vi "Main.vi"(11 "Module Admin":refnum<class "Delacor_lib_QMH_Module Admin.lvclass">) -> ()   [LabVIEW 2020, in "CML UI.lvlib"]
doc: "This template is based off of the Queued Message Handler design pattern and the Queued Message Handler project template that ships with LabVIEW.\n\nThe main difference is that the queue is private to this module and communication between modules is performed via Broadcast and Request events.\n\nRequest events are wrapped in public API methods and are handled in the Event Handling Loop (EHL) of this VI. Any module can register for Broadcast events sent by this module. The EHL generates messages based on user interface actions.\n\nThe Message Handling Loop (MHL) processes messages generated by the EHL, or by other messages. The messages are string values, so new messages can be added easily to the Message Cases case structure in the MHL. Each message cluster can also provide an optional value for Message Data, which is a variant that can be converted to whatever message-specific data is required.\n_____\nBased on DQMH Project Template 4.0.0.47.\n_____\nBased on DQMH Project Template 7.0.1.1316."
uses:
  CML UI.lvlib
  <vilib>/Delacor/Delacor QMH/Libraries/Module Admin_class/Delacor_lib_QMH_Module Admin.lvclass
  Module Data--cluster.ctl
  Configuration/Configuration--cluster.ctl
  Stop Argument--cluster.ctl
  <vilib>/Delacor/Delacor QMH/Libraries/Message Queue_class/Delacor_lib_QMH_Message Queue.lvclass/Delacor_lib_QMH_Message Queue.ctl
  <vilib>/Delacor/Delacor QMH/Libraries/Module Admin_class/Delacor_lib_QMH_Module Admin.lvclass/Delacor_lib_QMH_Module Admin.ctl
  Configuration/Configuration.lvclass
  Configuration/Configuration.lvclass/Configuration.ctl
  <vilib>/Delacor/Delacor QMH/Libraries/Message Queue_class/Delacor_lib_QMH_Enqueue Message (Single).vi
  <vilib>/Delacor/Delacor QMH/Libraries/Module Admin_class/Delacor_lib_QMH_Get External Launch.vi
  Configuration/Get Configuration.vi
  <vilib>/Delacor/Delacor QMH/Libraries/Message Queue_class/Delacor_lib_QMH_Message Queue.lvclass
  Settings Editor/Settings Editor.lvlib
  Acquisition/Acquisition.lvlib
  Logger/Logger.lvlib
  <vilib>/Peloton/Peloton Config/DCFG Framework/Peloton_lib_DCFG Framework.lvlib
  CML Shared/CML Shared.lvlib
  <vilib>/Peloton/Peloton Config/DCFG Framework/Configuration_class/Configuration.lvclass
panel:
  in  "About DQMH":bool
  out "Logger Running?":bool
  out "Settings Editor Running?":bool
  out "Acquisition Running?":bool
  out "Data":waveform(dbl)[](graph)
  out "Calibrated?":bool
  in  "Calibrate":bool
  in  "Settings":bool
  in  "Start":bool
  in  "Stop":bool
  out "error out":errorcluster
  out "Status":string
  out "version":string
  # "Continuous Measurement Data Logger"
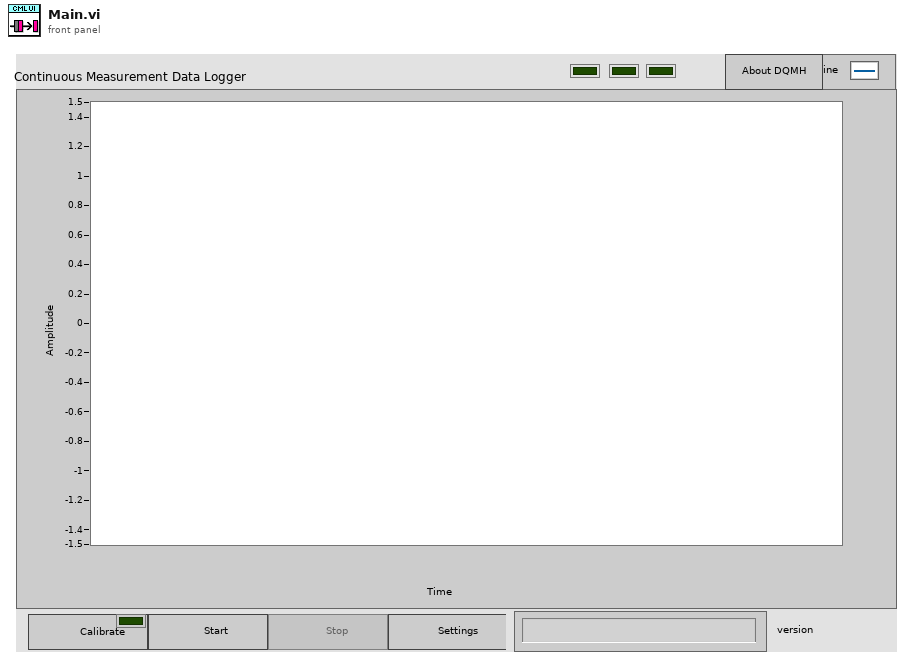
[diagram p1: front panel]
types:
  T1 = typedef "CML UI.lvlib/Request Events--cluster.ctl" = cluster{"Stop Module":refnum<user-event>, "Show Panel":refnum<user-event>, "Hide Panel":refnum<user-event>, "Get Module Execution Status":refnum<user-event>, "Show Diagram":refnum<user-event>}
  T2 = typedef "Settings Editor.lvlib/Broadcast Events--cluster.ctl" = cluster{"Module Did Init":refnum<user-event>, "Status Updated":refnum<user-event>, "Error Reported":refnum<user-event>, "Module Did Stop":refnum<user-event>, "Update Module Execution Status":refnum<user-event>, "Application Settings Updated":refnum<user-event>}
  T3 = typedef "Acquisition.lvlib/Broadcast Events--cluster.ctl" = cluster{"Module Did Init":refnum<user-event>, "Status Updated":refnum<user-event>, "Error Reported":refnum<user-event>, "Module Did Stop":refnum<user-event>, "Update Module Execution Status":refnum<user-event>, "Acquisition Started":refnum<user-event>, "Acquisition Stopped":refnum<user-event>, "Data Updated":refnum<user-event>, "Device Calibrated":refnum<user-event>}
  T4 = typedef "Logger.lvlib/Broadcast Events--cluster.ctl" = cluster{"Module Did Init":refnum<user-event>, "Status Updated":refnum<user-event>, "Error Reported":refnum<user-event>, "Module Did Stop":refnum<user-event>, "Update Module Execution Status":refnum<user-event>, "Logging Stopped":refnum<user-event>, "File Initialized":refnum<user-event>}
  T5 = typedef "Peloton_lib_DCFG Framework.lvlib/Broadcast Events--cluster.ctl" = cluster{"Module Did Init":refnum<user-event>, "Status Updated":refnum<user-event>, "Error Reported":refnum<user-event>, "Module Did Stop":refnum<user-event>, "Update Module Execution Status":refnum<user-event>, "View Changed":refnum<user-event>, "Main Window Closed":refnum<user-event>, "Configuration Committed":refnum<user-event>, "Configuration Canceled":refnum<user-event>, "Views List Updated":refnum<user-event>, "Config Folder Path Updated":refnum<user-event>}
  T6 = typedef "CML UI.lvlib/Module Data--cluster.ctl" = cluster{"Status":string, "Start Ref":refnum<vi>, "Settings Ref":refnum<vi>, "Stop Ref":refnum<vi>, "Status Ref":refnum<vi>, "Data Ref":refnum<vi>, "Configuration":T7}
  T7 = typedef "CML UI.lvlib/Configuration.lvclass/Configuration--cluster.ctl" = cluster{"test1":dbl, "test2":dbl}
  T8 = enum32{"invalid lock state", "Not Locked", "Locked (No Password)", "Password-protected"}
  T9 = typedef "CML UI.lvlib/Stop Argument--cluster.ctl" = cluster{"Origin":string, "Exit via Stop Module Req?":bool, "Wait for Module to stop?":bool}
  T10 = enum32{"Invalid", "Standard", "Closed", "Hidden", "Minimized", "Maximized"}
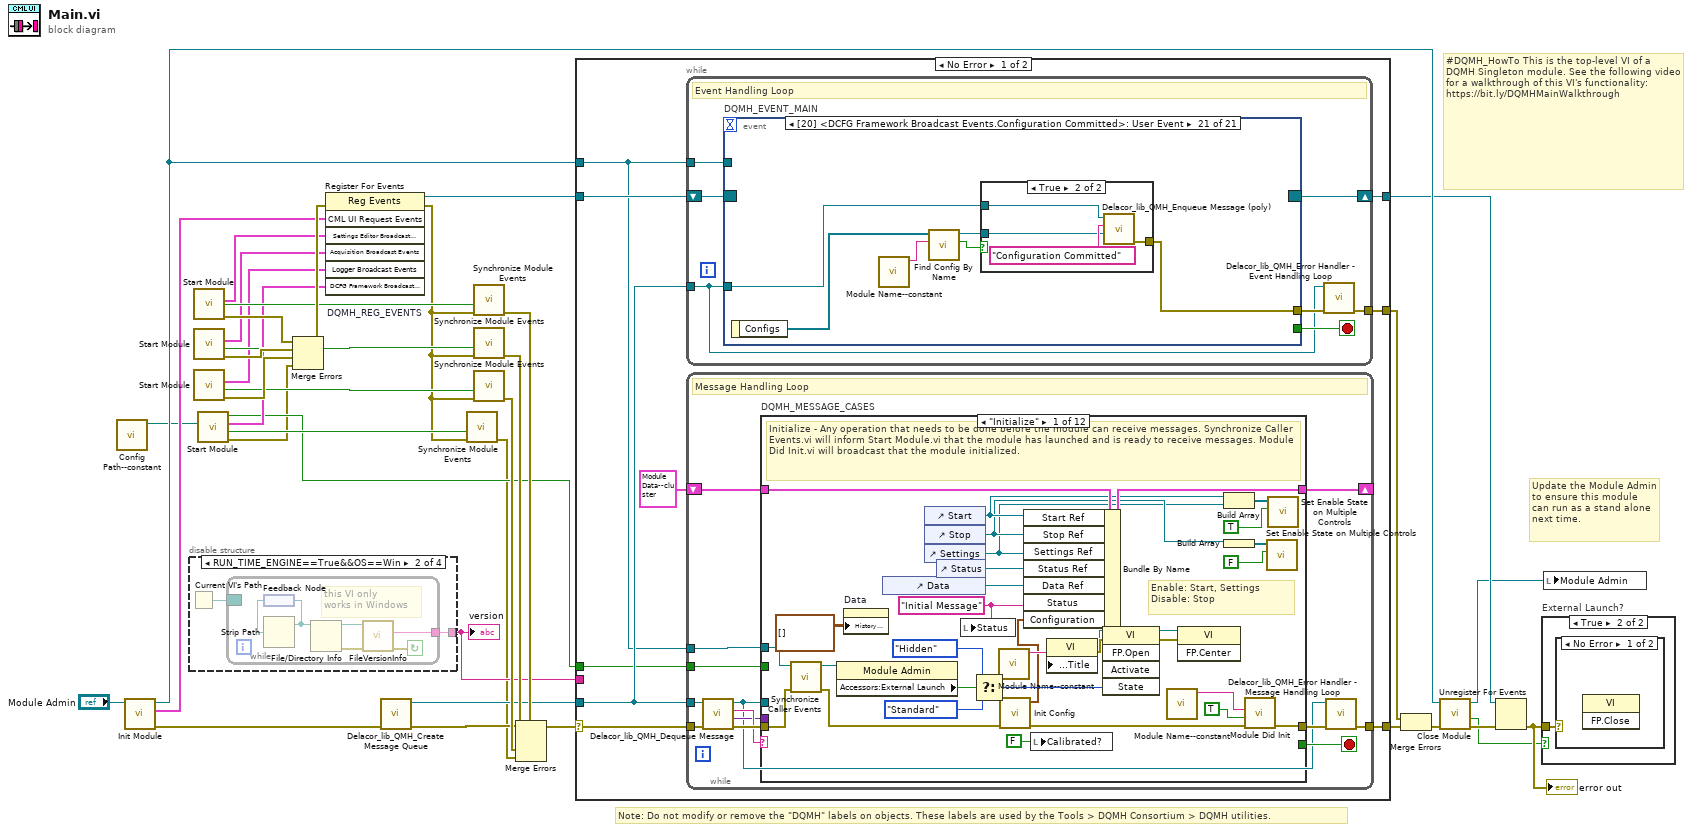
[diagram p0: block diagram]
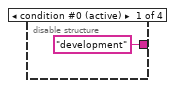
[diagram p2: hidden frame]
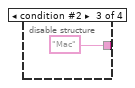
[diagram p3: hidden frame]
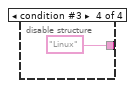
[diagram p4: hidden frame]
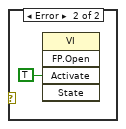
[diagram p6: hidden frame]
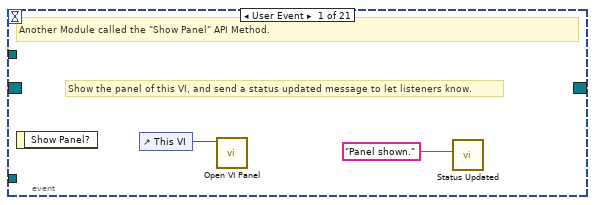
[diagram p7: hidden frame]
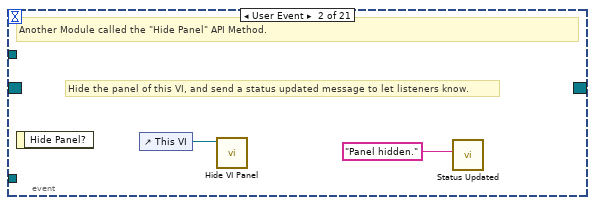
[diagram p8: hidden frame]
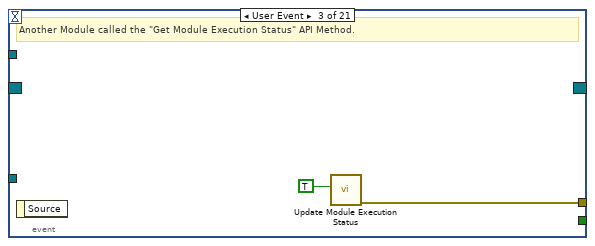
[diagram p9: hidden frame]
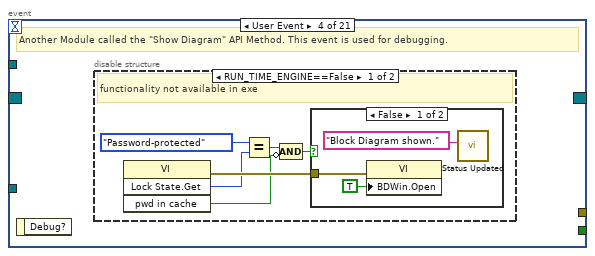
[diagram p10: hidden frame]
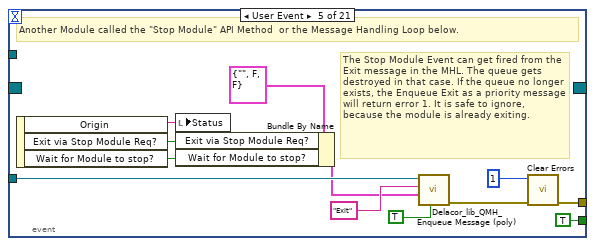
[diagram p13: hidden frame]
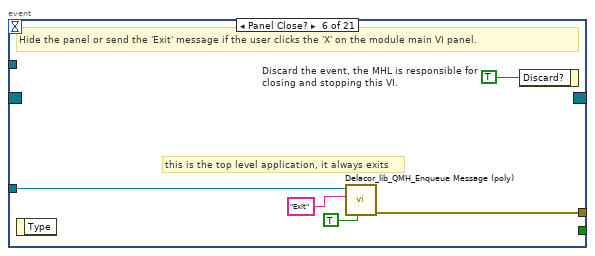
[diagram p14: hidden frame]
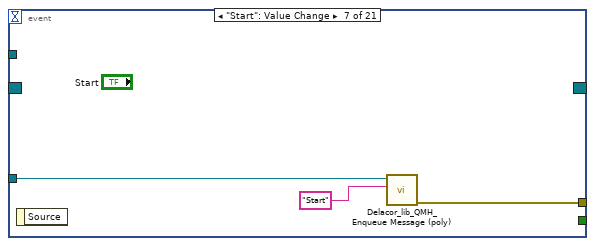
[diagram p15: hidden frame]
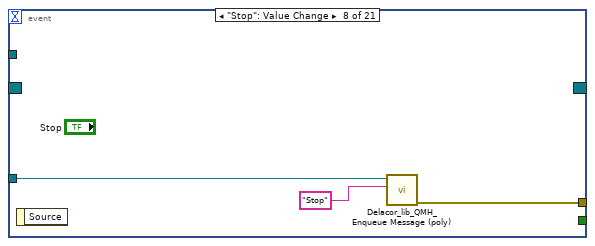
[diagram p16: hidden frame]
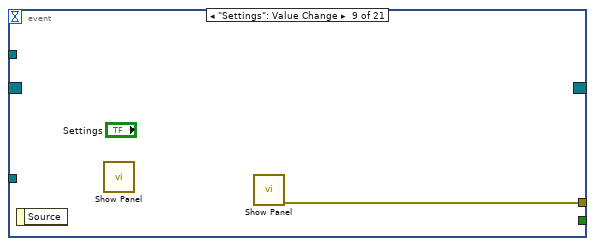
[diagram p17: hidden frame]
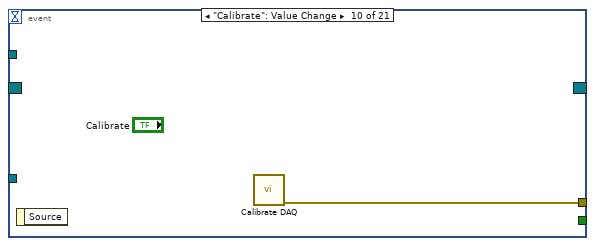
[diagram p18: hidden frame]
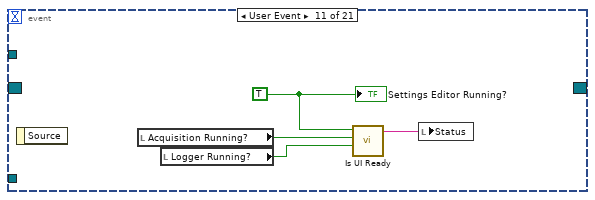
[diagram p19: hidden frame]
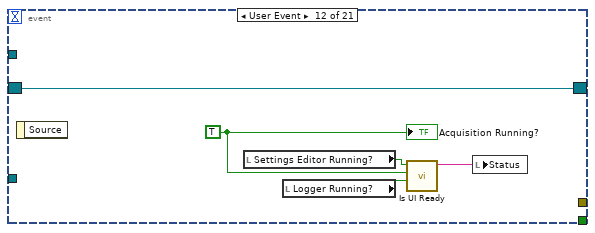
[diagram p20: hidden frame]
diagram:
  # "#DQMH_HowTo This is the top-level VI of a DQMH Singleton module. See the following video for a walkthrough of this VI's functionality: https://bit.ly/DQMHMainWalkthrough"
  # "Note: Do not modify or remove the \"DQMH\" labels on objects. These labels are used by the Tools > DQMH Consortium > DQMH utilities."
  # "Update the Module Admin to ensure this module can run as a stand alone next time."
  n1 = call "Config Path--constant.vi"() -> ("File Path"=w1:path)  [unwired: 11 in]
  n2 = call "Init Module.vi"("Singleton Module Admin in"="Module Admin") -> ("error out"=w35:errorcluster, "CML UI Request Events"=w19:T1, "Singleton Module Admin out"=w22:refnum<class "Delacor_lib_QMH_Module Admin.lvclass">)  [unwired: 8 in]
  n3 = disable-structure "Conditional Disable Structure" shown="RUN_TIME_ENGINE==True&&OS==Win" {
    disable-tunnel: ["development" w39 "Mac" "Linux"] -> w8
    frame condition #0 (active) {
    }
    frame condition #1 {
      n4 = Current VI's Path() -> (path=w40:path)
      n5 = while {
        border: w40 -> [_]
        tunnel: [w41] -> w39
        stop <- w45 continue-if-true
        # "this VI only \nworks in Windows"
        n6 = feedback #1() -> (w44:path)
        n7 = Strip Path(path=w44) -> (stripped path=w43:path)  [unwired: 1 out]
        n8 = feedback-in #1(w43) -> ()
        n9 = File/Directory Info(path=w43) -> (path out=w42:path, error out=w46:errorcluster)  [unwired: 1 in, 5 out]
        n10 = call <vilib>:"FileVersionInfo.vi"("error in (no error)"=w46, "Application Path in"=w42) -> ("error out"=w45:errorcluster, "File Version Info"=w41:string)  [unwired: 6 in, 2 out]
      }
    }
    frame condition #2 {
    }
    frame condition #3 {
    }
  }
  "version" <- w8
  n11 = call <vilib>:"Start Module.vi"() -> ("error out"=w26:errorcluster, "Wait for Event Sync?"=w14:bool, "Settings Editor Broadcast Events"=w13:T2)  [unwired: 8 in, 1 out]
  n12 = call <vilib>:"Start Module.vi"() -> ("error out"=w25:errorcluster, "Wait for Event Sync?"=w11:bool, "Acquisition Broadcast Events"=w12:T3)  [unwired: 8 in, 1 out]
  n13 = call <vilib>:"Start Module.vi"() -> ("error out"=w24:errorcluster, "Wait for Event Sync?"=w9:bool, "Logger Broadcast Events"=w10:T4)  [unwired: 8 in, 1 out]
  n14 = call <vilib>:"Start Module.vi"("Config Folder"=w1) -> ("error out"=w4:errorcluster, "Wait for Event Sync?"=w6:bool, "DCFG Framework Broadcast Events"=w7:T5, "Module Was Already Running?"=w5:bool)  [unwired: 7 in]
  n15 = Merge Errors(w26, w25, w24, w4) -> (w23:errorcluster)
  n16 = register-events "DQMH_REG_EVENTS"(error in=w23, w19, w13, w12, w10, w7) -> (reference out=w20:refnum<event-registration>, error out=w3:errorcluster)  [unwired: 1 in]
  n17 = call <vilib>:"Delacor_lib_QMH_Create Message Queue.vi"("error in"=w35) -> ("error out"=w30:errorcluster, "Message Queue"=w18:refnum<class "Delacor_lib_QMH_Message Queue.lvclass">)  [unwired: 9 in]
  n18 = call <vilib>:"Synchronize Module Events.vi"("error in (no error)"=w3, "Wait for Event Sync?"=w6) -> ("error out"=w2:errorcluster)  [unwired: 9 in]
  n19 = call <vilib>:"Synchronize Module Events.vi"("error in"=w3, "Wait for Event Sync?"=w14) -> ("error out"=w28:errorcluster)  [unwired: 9 in]
  n20 = call <vilib>:"Synchronize Module Events.vi"("error in"=w3, "Wait for Event Sync?"=w11) -> ("error out"=w27:errorcluster)  [unwired: 9 in]
  n21 = call <vilib>:"Synchronize Module Events.vi"("error in"=w3, "Wait for Event Sync?"=w9) -> ("error out"=w37:errorcluster)  [unwired: 9 in]
  n22 = Merge Errors(w30, w28, w27, w37, w2) -> (w29:errorcluster)
  n23 = case shown="No Error" w29 {
    selector: w29 -> [w55 w292]
    tunnel: [w57 w291] -> w36
    tunnel: [w54 w290] -> w21
    tunnel: w20 -> [w52 w290]
    tunnel: w18 -> [w51 w283]
    tunnel: [w56 _] -> w33
    tunnel: w22 -> [w50 w286]
    tunnel: w8 -> [_ _]
    tunnel: w5 -> [w49 w282]
    frame No Error {
      n24 = while {
        tunnel: w51 -> [w58]
        shift-right: [w61] -> w54
        shift-left: w52 -> [w62]
        tunnel: [w63] -> w56
        tunnel: w50 -> [w59]
        stop <- w60 stop-if-true
        # "Event Handling Loop"
        n25 = event "DQMH_EVENT_MAIN" shown="[20] <DCFG Framework Broadcast Events.Configuration Committed>: User Event" {
          selector: w62 -> [_ _ _ _ _ _ _ _ _ _ _ w113 _ _ _ _ _ _ _ _ _]
          dyn-events: [_ _ _ _ _ _ _ _ _ _ _ w113 _ _ _ _ _ _ _ _ _] -> w61
          timeout: _ -> [_ _ _ _ _ _ _ _ _ _ _ _ _ _ _ _ _ _ _ _ _]
          tunnel: [_ _ _ _ TRUE ("Discard?") _ _ _ _ _ _ _ _ _ _ _ _ _ _ _ _] -> w60
          tunnel: w58 -> [_ _ _ _ w87 w94 w97 w100 _ _ _ _ _ _ _ w125 w127 _ _ _ w134]
          tunnel: [_ _ w70 _ w90 w96 w99 w102 w103 w104 _ _ _ _ w123 _ _ _ _ w130 w136] -> w64
          tunnel: w59 -> [_ _ _ _ _ _ _ _ _ _ _ _ _ _ _ _ _ _ _ _ _]
          event User Event {
            # "Show the panel of this VI, and send a status updated message to let listeners know."
            # "Another Module called the \"Show Panel\" API Method."
            n26 = event-data() -> ()  [unwired: 1 in, 1 out]
            n27 = control-ref of="This VI"() -> (w66:refnum<vi>)
            n28 = call "Open VI Panel.vi"("VI"=w66) -> ()  [unwired: 10 in, 1 out]
            n29 = call "Status Updated.vi"("Status"="Panel shown." ("format string")) -> ()  [unwired: 10 in, 1 out]
          }
          event User Event {
            # "Hide the panel of this VI, and send a status updated message to let listeners know."
            # "Another Module called the \"Hide Panel\" API Method."
            n30 = event-data() -> ()  [unwired: 1 in, 1 out]
            n31 = control-ref of="This VI"() -> (w68:refnum<vi>)
            n32 = call "Hide VI Panel.vi"("VI"=w68) -> ()  [unwired: 10 in, 1 out]
            n33 = call "Status Updated.vi"("Status"="Panel hidden." ("format string")) -> ()  [unwired: 10 in, 1 out]
          }
          event User Event {
            # "Another Module called the \"Get Module Execution Status\" API Method."
            n34 = event-data() -> ()  [unwired: 1 in, 1 out]
            n35 = call "Update Module Execution Status.vi"("Running?"=TRUE) -> ("error out"=w70:errorcluster)  [unwired: 10 in]
          }
          event User Event {
            # "Another Module called the \"Show Diagram\" API Method. This event is used for debugging."
            n36 = event-data() -> ()  [unwired: 1 in, 1 out]
            n37 = disable-structure shown="RUN_TIME_ENGINE==False" {
              frame condition #0 (active) {
                # "functionality not available in exe"
                n38 = invoke on="Invoke Node" class="VI" method="Lock State.Get"() -> (error out=w76:errorcluster, "Get Lock State"=w75:T8, "pwd in cache"=w72:bool)  [unwired: 4 in, 1 out]
                n39 = Equal?(x=T8."Password-protected", y=w75) -> (x = y?=w73:bool)
                n40 = Compound Arithmetic op=AND(w73, invert w72) -> (w71:bool)
                n41 = case shown="False" w71 {
                  tunnel: w76 -> [w79 _]
                  frame False {
                    n42 = property on="Property Node" class="VI"(error in=w79, "BDWin.Open"=TRUE ("Block Diagram Window:Open")) -> ()  [unwired: 1 in, 2 out]
                    n43 = call "Status Updated.vi"("Status"="Block Diagram shown." ("format string")) -> ()  [unwired: 10 in, 1 out]
                  }
                  frame True {
                    # "Password-protected VI, and the password is not in the cache. Do not show the diagram."
                  }
                }
              }
              frame condition #1 {
              }
            }
          }
          event User Event {
            # "The Stop Module Event can get fired from the Exit message in the MHL. The queue gets destroyed in that case. If the queue no longer exists, the Enqueue Exit as a priority message will return error 1. It is safe to ignore, because the module is already exiting."
            # "Another Module called the \"Stop Module\" API Method  or the Message Handling Loop below."
            n44 = event-data() -> ("Origin"=w86:string, "Exit via Stop Module Req?"=w82:bool, "Wait for Module to stop?"=w81:bool)  [unwired: 1 in]
            n45 = local write "Status"(w86) -> ()
            n46 = Bundle By Name(cluster=T9 {"Origin"="", "Exit via Stop Module Req?"=FALSE, "Wait for Module to stop?"=FALSE} ("Stop Argument"), "Exit via Stop Module Req?"=w82, "Wait for Module to stop?"=w81) -> (w80:T9)
            n47 = call-poly <vilib>:"Delacor_lib_QMH_Enqueue Message (poly).vi"("Priority Message? (F)"=TRUE, "Message Data"=w80, "Message"="Exit", "Message Queue in"=w87) -> ("error out"=w91:errorcluster)  [unwired: 6 in, 1 out]
            n48 = call <vilib>:"Clear Errors.vi"("error in (no error)"=w91, "specific error code to clear (0: all)"=1) -> ("error out"=w90:errorcluster)  [unwired: 4 in, 1 out]
          }
          event Panel Close? {
            w95 = TRUE  # Discard the event, the MHL is responsible for closing and stopping this VI.
            # "this is the top level application, it always exits"
            # "Hide the panel or send the 'Exit' message if the user clicks the 'X' on the module main VI panel."
            n49 = event-data() -> ()  [unwired: 1 in, 1 out]
            n50 = call-poly <vilib>:"Delacor_lib_QMH_Enqueue Message (poly).vi"("Priority Message? (F)"=TRUE, "Message"="Exit", "Message Queue in"=w94) -> ("error out"=w96:errorcluster)  [unwired: 7 in, 1 out]
            n51 = event-data ("Event Filter Node")("Discard?"=w95) -> ()  [unwired: 1 in, 1 out]
          }
          event "Start": Value Change {
            n52 = event-data() -> ()  [unwired: 1 in, 1 out]
            n53 = call-poly <vilib>:"Delacor_lib_QMH_Enqueue Message (poly).vi"("Message"="Start", "Message Queue in"=w97) -> ("error out"=w99:errorcluster)  [unwired: 8 in, 1 out]
          }
          event "Stop": Value Change {
            n54 = event-data() -> ()  [unwired: 1 in, 1 out]
            n55 = call-poly <vilib>:"Delacor_lib_QMH_Enqueue Message (poly).vi"("Message"="Stop", "Message Queue in"=w100) -> ("error out"=w102:errorcluster)  [unwired: 8 in, 1 out]
          }
          event "Settings": Value Change {
            n56 = event-data() -> ()  [unwired: 1 in, 1 out]
            n57 = call <vilib>:"Show Panel.vi"() -> ()  [unwired: 11 in, 1 out]
            n58 = call <vilib>:"Show Panel.vi"() -> ("error out"=w103:errorcluster)  [unwired: 11 in]
          }
          event "Calibrate": Value Change {
            n59 = event-data() -> ()  [unwired: 1 in, 1 out]
            n60 = call "Calibrate DAQ.vi"() -> ("error out"=w104:errorcluster)  [unwired: 11 in]
          }
          event User Event {
            w106 = TRUE ("Settings Editor Running?")
            n61 = event-data() -> ()  [unwired: 1 in, 1 out]
            n62 = local read "Acquisition Running?"() -> (w108:bool)
            n63 = local read "Logger Running?"() -> (w107:bool)
            n64 = call "Is UI Ready.vi"("Logger Running?"=w107, "Acquisition Running?"=w108, "Settings Editor Running?"=w106) -> ("Status"=w105:string)  [unwired: 8 in]
            n65 = local write "Status"(w105) -> ()
            "Settings Editor Running?" <- w106
          }
          event User Event {
            w111 = TRUE ("Acquisition Running?")
            n66 = event-data() -> ()  [unwired: 1 in, 1 out]
            n67 = local read "Settings Editor Running?"() -> (w110:bool)
            n68 = local read "Logger Running?"() -> (w109:bool)
            n69 = call "Is UI Ready.vi"("Logger Running?"=w109, "Acquisition Running?"=w111, "Settings Editor Running?"=w110) -> ("Status"=w112:string)  [unwired: 8 in]
            n70 = local write "Status"(w112) -> ()
            "Acquisition Running?" <- w111
          }
          event User Event {
            w116 = TRUE ("Logger Running?")
            n71 = event-data() -> ()  [unwired: 1 in, 1 out]
            n72 = local read "Settings Editor Running?"() -> (w115:bool)
            n73 = local read "Acquisition Running?"() -> (w114:bool)
            n74 = call "Is UI Ready.vi"("Logger Running?"=w116, "Acquisition Running?"=w114, "Settings Editor Running?"=w115) -> ("Status"=w117:string)  [unwired: 8 in]
            n75 = local write "Status"(w117) -> ()
            "Logger Running?" <- w116
          }
          event User Event {
            n76 = event-data() -> ("Status"=w118:string)  [unwired: 1 in]
            "Status" <- w118
            n77 = call "Status Updated.vi"("Status"=w118) -> ()  [unwired: 10 in, 1 out]
          }
          event User Event {
            n78 = event-data() -> ("Error"=w123:errorcluster, "Module Name"=w121:string)  [unwired: 1 in]
            n79 = Unbundle By Name(w123) -> ("code"=w122:i32)
            n80 = Format Into String(format string="Error %d at %s", w122, w121) -> (resulting string=w120:string)  [unwired: 2 in, 1 out]
            n81 = local write "Status"(w120) -> ()
          }
          event User Event {
            n82 = event-data() -> ()  [unwired: 1 in, 1 out]
            n83 = call-poly <vilib>:"Delacor_lib_QMH_Enqueue Message (poly).vi"("Message"="Acquisition Started Interlocks", "Message Queue in"=w125) -> ()  [unwired: 8 in, 2 out]
          }
          event User Event {
            n84 = event-data() -> ()  [unwired: 1 in, 1 out]
            n85 = call-poly <vilib>:"Delacor_lib_QMH_Enqueue Message (poly).vi"("Message"="Acquisition Stopped Interlocks", "Message Queue in"=w127) -> ()  [unwired: 8 in, 2 out]
          }
          event User Event {
            n86 = event-data() -> ("Graph Data"=→"Data":waveform(dbl)[])  [unwired: 1 in]
          }
          event User Event {
            n87 = event-data() -> ()  [unwired: 1 in, 1 out]
            "Calibrated?" <- TRUE ("Calibrated?")
          }
          event "About DQMH": Value Change {
            # "Display the About DQMH box"
            n88 = event-data() -> ()  [unwired: 1 in, 1 out]
            n89 = call <vilib>:"DQMH_About Box.vi"() -> ("error out"=w130:errorcluster)  [unwired: 11 in]
          }
          event User Event {
            n90 = event-data() -> ("Configs"=w135:refnum<class "Configuration.lvclass">[])  [unwired: 1 in]
            n91 = call "Module Name--constant.vi"() -> ("Module Name"=w133:string)  [unwired: 11 in]
            n92 = call <vilib>:"Find Config By Name.vi"("Config Name"=w133, "All Config Classes"=w135) -> ("Found"=w132:bool, "Configuration"=w131:refnum<class "Configuration.lvclass">)  [unwired: 6 in, 2 out]
            n93 = case shown="True" w132 {
              tunnel: w134 -> [_ w139]
              tunnel: [_ w140] -> w136
              tunnel: w131 -> [_ w137]
              frame False {
              }
              frame True {
                n94 = call-poly <vilib>:"Delacor_lib_QMH_Enqueue Message (poly).vi"("Message Data"=w137, "Message"="Configuration Committed", "Message Queue in"=w139) -> ("error out"=w140:errorcluster)  [unwired: 7 in, 1 out]
              }
            }
          }
        }
        n95 = call-dynamic "Delacor_lib_QMH_Error Handler - Event Handling Loop.vi"("error in"=w64, "Message Queue in"=w58) -> ("dup error in"=w63:errorcluster)  [unwired: 8 in, 1 out]
      }
      n96 = while {
        tunnel: w51 -> [w144]
        shift-right: [w148] -> _
        shift-left: T6 {"Status"="", "Start Ref"=refnum, "Settings Ref"=refnum, "Stop Ref"=refnum, "Status Ref"=refnum, "Data Ref"=refnum, "Configuration"={"test1"=0.0, "test2"=0.0}} ("Data Cluster") -> [w149]
        tunnel: w55 -> [w152]
        tunnel: [w150] -> w57
        tunnel: w50 -> [w142]
        tunnel: w49 -> [w141]
        stop <- w147 stop-if-true
        # "Message Handling Loop"
        n97 = call-dynamic "Delacor_lib_QMH_Dequeue Message.vi"("error in"=w152, "Message Queue in"=w144) -> ("error out"=w151:errorcluster, "Message Data"=w145:variant, "Message"=w146:string, "Message Queue out"=w143:refnum<class "Delacor_lib_QMH_Message Queue.lvclass">)  [unwired: 6 in]
        n98 = case "DQMH_MESSAGE_CASES" shown="\"Initialize\"" w146 {
          selector: w146 -> [_ _ _ _ _ _ _ _ _ _ w268 _]
          tunnel: w143 -> [_ _ _ _ _ _ _ _ w221 w249 _ _]
          tunnel: w151 -> [w183 w187 w190 w200 w203 w213 w216 w218 w229 w257 w271 w280]
          tunnel: [w182 w187 w189 w200 w202 w213 w215 w218 w225 w250 w272 w277] -> w153
          tunnel: w149 -> [w173 w186 w188 w192 w201 w205 w214 w217 w223 w248 w269 w279]
          tunnel: [w165 w186 w188 w192 w201 w205 w214 w217 w223 w248 w269 w278] -> w148
          tunnel: [_ _ _ _ _ _ _ _ _ w247 _ _] -> w147
          tunnel: w145 -> [_ _ _ _ _ _ _ _ w222 w246 _ w276]
          tunnel: w142 -> [w174 _ _ _ _ _ _ _ w220 w241 _ _]
          tunnel: w141 -> [_ _ _ _ _ _ _ _ _ w237 _ _]
          frame "Initialize" {
            w168 = "Initial Message" ("Initial Message")
            # "Enable: Start, Settings\nDisable: Stop"
            # "Initialize - Any operation that needs to be done before the module can receive messages. Synchronize Caller Events.vi will inform Start Module.vi that the module has launched and is ready to receive messages. Module Did Init.vi will broadcast that the module initialized."
            n99 = call "Synchronize Caller Events.vi"("error in"=w183, "Singleton Module Admin in"=w174) -> ("error out"=w156:errorcluster, "Singleton Module Admin out"=w170:refnum<class "Delacor_lib_QMH_Module Admin.lvclass">)  [unwired: 8 in]
            n100 = property on="Property Node" class="Module Admin"(reference=w170) -> ("Accessors:External Launch"=w178:bool)  [unwired: 1 in, 2 out]
            n101 = property on="Data" class="WFChart (strict)"("History Data"=waveform(dbl)[][] []) -> ()  [unwired: 2 in, 2 out]
            n102 = control-ref of="Data"() -> (w166:refnum<vi>)
            n103 = control-ref of="Start"() -> (w159:refnum<vi>)
            n104 = control-ref of="Stop"() -> (w158:refnum<vi>)
            n105 = control-ref of="Settings"() -> (w157:refnum<vi>)
            n106 = control-ref of="Status"() -> (w167:refnum<vi>)
            n107 = local write "Status"(w168) -> ()
            n108 = Select(t=T10."Hidden" ("State"), s=w178, f=T10."Standard" ("State")) -> (s? t:f=w175:T10)
            n109 = call "Module Name--constant.vi"() -> ("Module Name"=w181:string)  [unwired: 11 in]
            n110 = call "Init Config.vi"("error in"=w156) -> ("error out"=w155:errorcluster, "Configuration"=w154:T7)  [unwired: 9 in]
            n111 = Bundle By Name(cluster=w173, "Start Ref"=w159, "Stop Ref"=w158, "Settings Ref"=w157, "Status Ref"=w167, "Data Ref"=w166, "Status"=w168, "Configuration"=w154) -> (w165:T6)
            n112 = local write "Calibrated?"(FALSE ("Calibrated?")) -> ()
            n113 = property on="Property Node" class="VI"("Front Panel.Title"=w181) -> (reference out=w180:refnum<vi>, error out=w185:errorcluster)  [unwired: 2 in]
            n114 = invoke on="Invoke Node" class="VI" method="FP.Open"(reference=w180, error in=w185, "State"=w175) -> (reference out=w179:refnum<vi>, error out=w184:errorcluster)  [unwired: 2 in, 3 out]
            n115 = call "Module Name--constant.vi"() -> ("Module Name"=w171:string)  [unwired: 11 in]
            n116 = invoke on="Invoke Node" class="VI" method="FP.Center"(reference=w179, error in=w184) -> ()  [unwired: 1 in, 3 out]
            n117 = Build Array(w159, w157) -> (w164:refnum<vi>[])
            n118 = Build Array(w158) -> (w162:refnum<vi>[])
            n119 = call "Module Did Init.vi"("error in"=w155, "Initialized?"=TRUE, "Origin"=w171) -> ("error out"=w182:errorcluster)  [unwired: 8 in]
            n120 = call "Set Enable State on Multiple Controls.vi"("Enable?"=FALSE, "Controls"=w162) -> ()  [unwired: 10 in]
            n121 = call "Set Enable State on Multiple Controls.vi"("Enable?"=TRUE, "Controls"=w164) -> ()  [unwired: 10 in]
          }
          frame "---Module Specific---" {
            # "Separator -- The following cases handle messages specific to this Module."
          }
          frame "Start" {
            # "End user pressed Start button. Need to request for Acquisition to start acquiring and for Logger to start logging."
            n122 = call "Initialize File.vi"("error in"=w190) -> ("error out"=w191:errorcluster)  [unwired: 8 in, 2 out]
            n123 = call "Start Acquiring.vi"("error in"=w191) -> ("error out"=w189:errorcluster)  [unwired: 8 in, 2 out]
          }
          frame "Acquisition Started Interlocks" {
            # "Enable: Stop\nDisable: Start, Settings"
            n124 = Unbundle By Name(w192) -> ("Stop Ref"=w199:refnum<vi>, "Start Ref"=w194:refnum<vi>, "Settings Ref"=w193:refnum<vi>)
            n125 = Build Array(w199) -> (w198:refnum<vi>[])
            n126 = Build Array(w194, w193) -> (w195:refnum<vi>[])
            n127 = call "Set Enable State on Multiple Controls.vi"("Enable?"=TRUE, "Controls"=w198) -> ()  [unwired: 10 in]
            n128 = call "Set Enable State on Multiple Controls.vi"("Enable?"=FALSE, "Controls"=w195) -> ()  [unwired: 10 in]
          }
          frame "Stop" {
            # "End user pressed Stop button. Need to request for Acquisition to stop acquiring and for Logger to stop logging."
            n129 = call "Stop Acquiring.vi"("error in"=w203) -> ("error out"=w204:errorcluster)  [unwired: 10 in]
            n130 = call "Stop Logging.vi"("error in"=w204) -> ("error out"=w202:errorcluster)  [unwired: 10 in]
          }
          frame "Acquisition Stopped Interlocks" {
            # "Enable: Start, Settings\nDisable: Stop"
            n131 = Unbundle By Name(w205) -> ("Stop Ref"=w210:refnum<vi>, "Start Ref"=w209:refnum<vi>, "Settings Ref"=w208:refnum<vi>)
            n132 = Build Array(w210) -> (w212:refnum<vi>[])
            n133 = Build Array(w209, w208) -> (w207:refnum<vi>[])
            n134 = call "Set Enable State on Multiple Controls.vi"("Enable?"=FALSE, "Controls"=w212) -> ()  [unwired: 10 in]
            n135 = call "Set Enable State on Multiple Controls.vi"("Enable?"=TRUE, "Controls"=w207) -> ()  [unwired: 10 in]
          }
          frame "---Copy This Frame---" {
            # "Duplicate this frame when creating new messages.  Change this comment in the duplicated frame to describe this message."
            n136 = Merge Errors(w216) -> (w215:errorcluster)
          }
          frame "---Exit and Error Handling---" {
            # "Separator - The following cases handle errors and exit messages."
          }
          frame "Error" {
            # "Error - Check the error message data and respond accordingly. This message is sent by the \"Error Handler\" VIs at the end of each loop in this application."
            n137 = property on="Property Node" class="Module Admin"(reference=w220) -> ("Accessors:External Launch"=w219:bool)  [unwired: 1 in, 2 out]
            n138 = Variant To Data(error in=w229, type=errorcluster {"status"=FALSE, "code"=0, "source"=""} ("error constant"), Variant=w222) -> (data=w224:errorcluster, error out=w227:errorcluster)
            n139 = local write "error out"(w224) -> ()
            n140 = call "Error Reported.vi"("Error"=w224) -> ()  [unwired: 10 in, 1 out]
            n141 = case shown="False" w219 {
              tunnel: [w234 _] -> w226
              tunnel: w221 -> [w232 _]
              tunnel: w224 -> [w233 _]
              frame False {
                n142 = disable-structure shown="Default" {
                  disable-tunnel: w233 -> [w235 _]
                  frame condition #0 (active) {
                    # "If the module is running standalone, then pop up an error dialog and call the \"Exit\" message."
                    n143 = call <vilib>:"Simple Error Handler.vi"("error in (no error)"=w235) -> ()  [unwired: 4 in, 5 out]
                  }
                  frame condition #1 {
                    # "To prevent the Simple Error Handler VI from being loaded (e.g. when deploying to a Real-Time target), add the Conditional Disable Symbol \"DQMH_Disable_SEH\" to your project and set it to TRUE."
                  }
                }
                n144 = call-poly <vilib>:"Delacor_lib_QMH_Enqueue Message (poly).vi"("Priority Message? (F)"=TRUE, "Message"="Exit", "Message Queue in"=w232) -> ("error out"=w234:errorcluster)  [unwired: 7 in, 1 out]
              }
              frame True {
                # "If the module was launched externally, calling the Error Reported broadcast VI is the only action performed by the \"Error\" message. The module's caller can then process the error appropriately."
              }
            }
            n145 = Merge Errors(w227, w226) -> (w225:errorcluster)
          }
          frame "Exit" {
            w240 = TRUE ("Wait for Module to Stop? (F)")
            w247 = TRUE  # Stop the VI
            # "DAQ and LOG modules use the settings editor. CML UI module waits for both modules to completely stop before stopping the settings editor."
            # "Release the message queue reference"
            # "Exit - Exit the application."
            n146 = Variant To Data(error in=w257, type=T9 {"Origin"="", "Exit via Stop Module Req?"=FALSE, "Wait for Module to stop?"=FALSE} ("Stop Argument"), Variant=w246) -> (data=w243:T9, error out=w254:errorcluster)
            n147 = call "Destroy Config.vi"() -> ("error out"=w238:errorcluster)  [unwired: 11 in]
            n148 = call <vilib>:"Clear Errors.vi"("error in (no error)"=w254, "specific error code to clear (0: all)"=91 ("91: not all Exit messages will have an argument")) -> ("error out"=w256:errorcluster)  [unwired: 4 in, 1 out]
            n149 = case "DCFG_Stop_Case" shown="True" w237 {
              tunnel: w238 -> [w261 w262]
              tunnel: [w260 w262] -> w236
              frame False {
                n150 = call <vilib>:"Stop Module.vi"("error in (no error)"=w261) -> ("error out"=w260:errorcluster)  [unwired: 10 in]
              }
              frame True {
                # "Let DCFG Running if it was already running"
              }
            }
            n151 = control-ref of="This VI"() -> (w242:refnum<vi>)
            n152 = call "Module Name--constant.vi"() -> ("Module Name"=w239:string)  [unwired: 11 in]
            n153 = call "Handle Exit.vi"("Stop Argument"=w243, "Admin in"=w241, "VI reference"=w242) -> ("error out"=w253:errorcluster)  [unwired: 7 in, 1 out]
            n154 = call <vilib>:"Stop Module.vi"("Wait for Module to Stop? (F)"=w240, "Origin"=w239) -> ("error out"=w252:errorcluster)  [unwired: 9 in]
            n155 = call <vilib>:"Stop Module.vi"("Wait for Module to Stop? (F)"=w240, "Origin"=w239) -> ("error out"=w251:errorcluster)  [unwired: 9 in]
            n156 = call-dynamic "Delacor_lib_QMH_Release Message Queue.vi"("error in"=w256, "Message Queue"=w249) -> ("error out"=w255:errorcluster)  [unwired: 9 in]
            n157 = Merge Errors(w252, w251) -> (w258:errorcluster)
            n158 = Merge Errors(w236, w255, w253) -> (w250:errorcluster)
            n159 = call <vilib>:"Clear Errors.vi"("error in (no error)"=w258) -> ("error out"=w259:errorcluster)  [unwired: 5 in, 1 out]
            n160 = call "Error Reported.vi"("Error"=w250) -> ()  [unwired: 10 in, 1 out]
            n161 = call <vilib>:"Stop Module.vi"("error in"=w259, "Wait for Module to Stop? (F)"=w240, "Origin"=w239) -> ()  [unwired: 8 in, 1 out]
          }
          frame Default {
            # "'Default' case only runs if there is a message that isn't defined in any of the other cases.  Output a programming error."
            n162 = call "Module Name--constant.vi"() -> ("Module Name"=w267:string)  [unwired: 11 in]
            n163 = Format Into String(format string="The invalid message string \"%s\" was received in the Message Handling Loop for module \"%s\".", w268, w267) -> (resulting string=w265:string)  [unwired: 2 in, 1 out]
            n164 = call <vilib>:"Error Cluster From Error Code.vi"("show call chain? (False)"=TRUE, "error message (\"\")"=w265, "error code (0)"=1) -> ("error out"=w270:errorcluster)  [unwired: 6 in]
            n165 = Merge Errors(w271, w270) -> (w272:errorcluster)
          }
          frame "Configuration Committed" {
            w274 = refnum<class "Configuration.lvclass"> refnum  # Module_Config_Class
            n166 = Variant To Data(error in=w280, type=w274, Variant=w276) -> (data=w273:refnum<class "Configuration.lvclass">, error out=w277:errorcluster)
            n167 = property on="Property Node" class="Config"(reference=w273) -> ("Accessors:Configuration"=w275:T7)  [unwired: 1 in, 2 out]
            n168 = Bundle By Name(cluster=w279, "Configuration"=w275) -> (w278:T6)
          }
        }
        n169 = call-dynamic "Delacor_lib_QMH_Error Handler - Message Handling Loop.vi"("error in"=w153, "Message Queue in"=w143) -> ("dup error in"=w150:errorcluster)  [unwired: 8 in, 1 out]
      }
    }
    frame Error {
      w285 = TRUE ("Wait for Module to Stop? (F)")
      # "Synchronize Caller Events.vi will inform Start Module.vi that the module has launched and will let the code calling Start Module.vi register for broadcasts and would permit the caller receive the broadcast that an error occurred at launch time."
      n170 = call-dynamic "Delacor_lib_QMH_Release Message Queue.vi"("error in"=w292, "Message Queue"=w283) -> ("error out"=w291:errorcluster)  [unwired: 9 in]
      n171 = call "Synchronize Caller Events.vi"("Singleton Module Admin in"=w286) -> ("error out"=w293:errorcluster)  [unwired: 9 in, 1 out]
      n172 = case "DCFG_Stop_Case" shown="True" w282 {
        tunnel: [w295 _] -> w281
        frame False {
          n173 = call <vilib>:"Stop Module.vi"() -> ("error out"=w295:errorcluster)  [unwired: 11 in]
        }
        frame True {
          # "Let DCFG Running if it was already running"
        }
      }
      n174 = call "Module Name--constant.vi"() -> ("Module Name"=w289:string)  [unwired: 11 in]
      n175 = call "Module Name--constant.vi"() -> ("Module Name"=w284:string)  [unwired: 11 in]
      n176 = call <vilib>:"Stop Module.vi"("Wait for Module to Stop? (F)"=w285, "Origin"=w284) -> ()  [unwired: 9 in, 1 out]
      n177 = call <vilib>:"Stop Module.vi"("Wait for Module to Stop? (F)"=w285, "Origin"=w284) -> ()  [unwired: 9 in, 1 out]
      n178 = call <vilib>:"Stop Module.vi"("Wait for Module to Stop? (F)"=w285, "Origin"=w284) -> ()  [unwired: 9 in, 1 out]
      n179 = Format Into String(format string="An error occurred during initialization. %s is no longer running.", w289) -> (resulting string=w287:string)  [unwired: 2 in, 1 out]
      n180 = Merge Errors(w291, w293, w281) -> (w294:errorcluster)
      n181 = call "Error Reported.vi"("Additional Information"=w287, "Error"=w294) -> ()  [unwired: 9 in, 1 out]
    }
  }
  n182 = Merge Errors(w33, w36) -> (w32:errorcluster)
  n183 = call "Close Module.vi"("error in"=w32, "Module Admin in"=w22) -> ("error out"=w34:errorcluster, "External Launch"=w15:bool, "Module Admin out"=w16:refnum<class "Delacor_lib_QMH_Module Admin.lvclass">)  [unwired: 7 in]
  n184 = Unregister For Events(event registration refnum=w21, error in=w34) -> (error out=w31:errorcluster)
  "error out" <- w31
  n185 = case "External Launch?" shown="True" w15 {
    tunnel: w31 -> [_ w296]
    frame False {
    }
    frame True {
      n186 = case shown="No Error" w296 {
        frame No Error {
          n187 = invoke on="Invoke Node" class="VI" method="FP.Close"() -> ()  [unwired: 3 in, 3 out]
        }
        frame Error {
          n188 = invoke on="Invoke Node" class="VI" method="FP.Open"("Activate"=TRUE ("Activate?")) -> ()  [unwired: 4 in, 5 out]
        }
      }
    }
  }
  n189 = local write "Module Admin"(w16) -> ()
